vi "StartTopicServer.vi"(2 "Baxter in":T1, 3 "Registration":enum16{"Register", "Unregister"}(ring)) -> (0 "Baxter out":T1)   [LabVIEW 2010]
uses:
  <userlib>/ROSforLV_0.1/ROS/Code/SubVIs/_ROSControl.ctl
  <userlib>/ROSforLV_0.1/ROS/Code/SubVIs/_ROSDirection.ctl
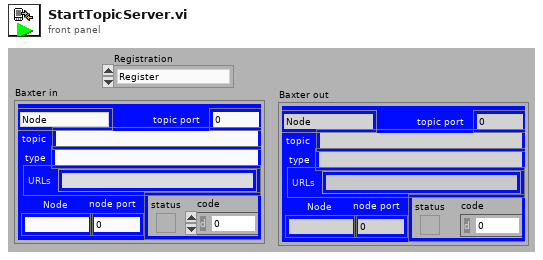
[diagram p1: front panel]
types:
  T1 = typedef "_ROSControl.ctl" = cluster{"topic port":u16, "Node":string, "topic":string, "type":string, "node port":u32, "error ":errorcluster, "Direction":T2, "APIs":string[]}
  T2 = typedef "_ROSDirection.ctl" = enum16{"Node", "Publisher", "Subscriber", "Service Client"}
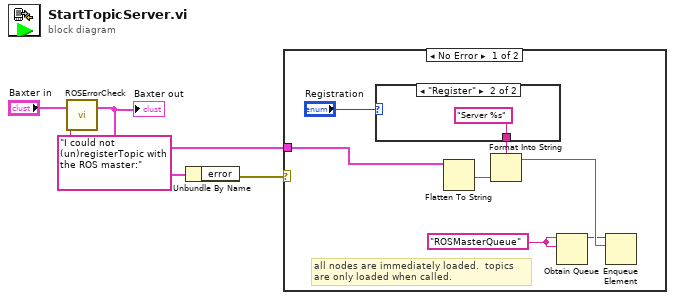
[diagram p0: block diagram]
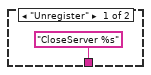
[diagram p2: hidden frame]
diagram:
  n1 = call <userlib>:"ROSErrorCheck.vi"("message"="I could not (un)registerTopic with the ROS master:", "ROS in"="Baxter in") -> ("ROS out"=w1:T1)  [unwired: 1 in]
  "Baxter out" <- w1
  n2 = Unbundle By Name(w1) -> ("error"=w4:errorcluster)
  n3 = case shown="No Error" w4 {
    tunnel: w1 -> [w6 _]
    frame No Error {
      w7 = "ROSMasterQueue" ("name (unnamed)")
      # "all nodes are immediately loaded.  topics\nare only loaded when called."
      n4 = case shown="\"Register\"" "Registration" {
        tunnel: ["CloseServer %s" ("format string") "Server %s" ("format string")] -> w10
        frame "Unregister" {
        }
        frame "Register" {
        }
      }
      n5 = Flatten To String(anything=w6) -> (data string=w5:string)  [unwired: 3 in, 2 out]
      n6 = Format Into String(format string=w10, w5) -> (resulting string=w9:string)  [unwired: 2 in, 1 out]
      n7 = Obtain Queue(name (unnamed)=w7, element data type=w7) -> (queue out=w8:refnum<queue>)  [unwired: 3 in, 2 out]
      n8 = Enqueue Element(queue=w8, element=w9) -> ()  [unwired: 2 in, 3 out]
    }
    frame Error {
    }
  }
